vi "DELETE REASON.vi"(8 "error in (no error)":errorcluster, 11 "connection reference":T1) -> (0 "error out":errorcluster, 3 "connection reference out":T1)   [LabVIEW 2017]
uses:
  <vilib>/addons/database/Connection.llb/Conn ObjectReference.ctl
  <vilib>/addons/database/NI_Database_API.lvlib
panel:
  in  "CANCEL":bool
  in  "Select Serial Number":string(combo)
  in  "DELETE":bool
  # "Delete Reason"
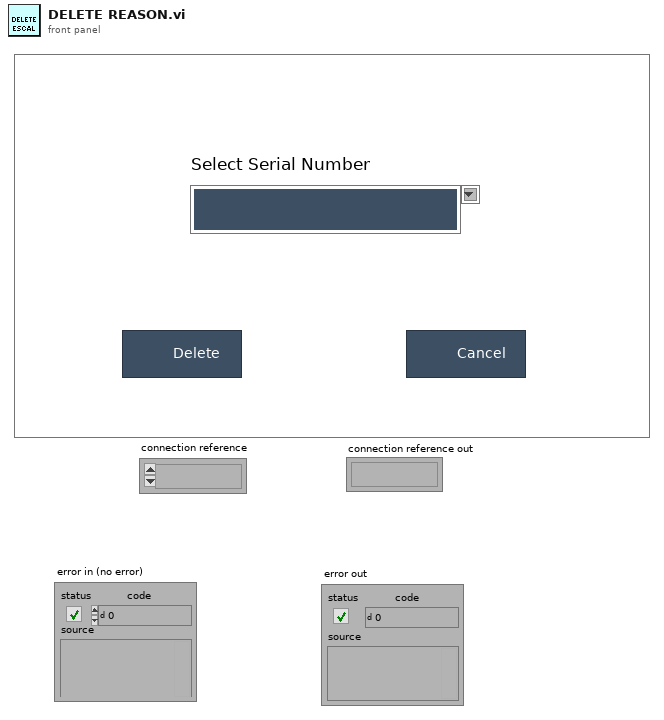
[diagram p1: front panel]
types:
  T1 = typedef "NI_Database_API.lvlib/Conn ObjectReference.ctl" = refnum<k1>
  T2 = enum32{"invalid app kind", "Development System", "Run Time System", "Student Edition", "Embedded LabVIEW", "Evaluation", "Custom"}
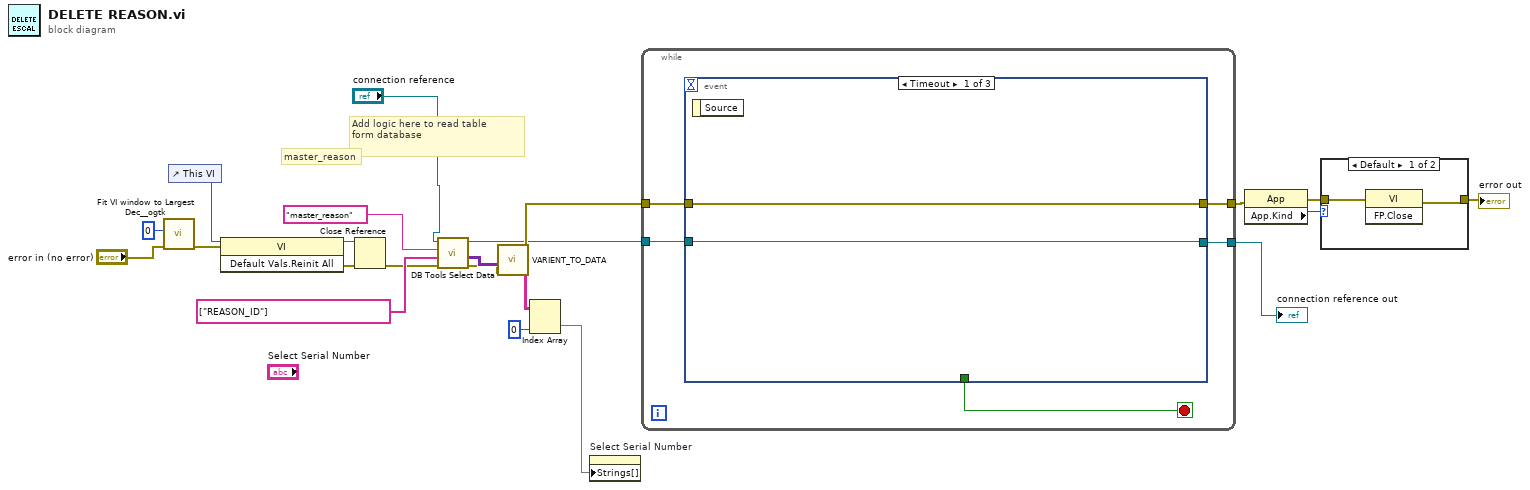
[diagram p0: block diagram]
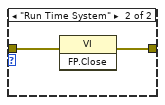
[diagram p2: hidden frame]
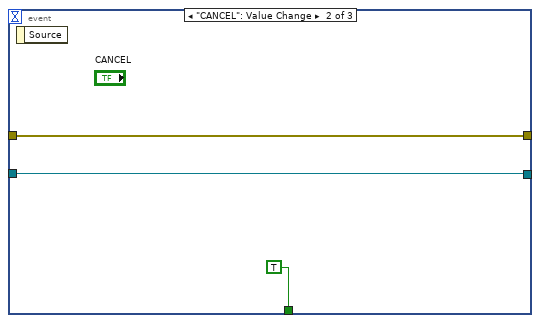
[diagram p3: hidden frame]
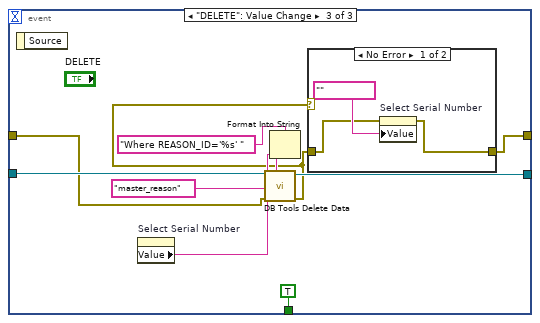
[diagram p4: hidden frame]
diagram:
  # "master_reason"
  # "Add logic here to read table\nform database"
  n1 = call <userlib>:"Fit VI window to Largest Dec__ogtk.vi"("error in (no error)"="error in (no error)", "border spacing (2 px)"=0) -> ("error out"=w2:errorcluster)  [unwired: 4 in, 1 out]
  n2 = control-ref of="This VI"() -> (w22:refnum<vi>)
  n3 = invoke class="VI" method="Default Vals.Reinit All"(reference=w22, error in=w2) -> (reference out=w20:refnum<vi>, error out=w21:errorcluster)  [unwired: 1 in, 1 out]
  n4 = Close Reference(reference=w20, error in (no error)=w21) -> (error out=w4:errorcluster)
  n5 = call <vilib>:"DB Tools Select Data.vi"("error in (no error)"=w4, "columns"=string[] ["REASON_ID"], "table"="master_reason", "connection reference"="connection reference") -> ("error out"=w14:errorcluster, "data"=w15:variant[][], "connection reference out"=w7:T1)  [unwired: 2 in]
  n6 = call "VARIENT_TO_DATA.vi"("data"=w15, "error in (no error)"=w14) -> ("Table"=w10:string[][], "error out"=w11:errorcluster)  [unwired: 7 in]
  n7 = Index Array(array=w10, index (col)=0 ("disabled index (col)")) -> (element=w8:string[])  [unwired: 1 in]
  n8 = property on="Select Serial Number" class="CmbBox"("Strings[]"=w8) -> ()  [unwired: 2 in, 2 out]
  n9 = while {
    tunnel: w11 -> [w27]
    tunnel: [w26] -> w16
    tunnel: w7 -> [w25]
    tunnel: [w24] -> w6
    stop <- w23 stop-if-true
    n10 = event shown="[0] Timeout" {
      selector: _ -> [_ _ _]
      dyn-events: _ -> [_ _ _]
      timeout: _ -> [_ _ _]
      tunnel: w27 -> [w29 w30 w41]
      tunnel: [w29 w30 w35] -> w26
      tunnel: w25 -> [w28 w31 w42]
      tunnel: [w28 w31 w40] -> w24
      tunnel: [_ TRUE TRUE] -> w23
      event Timeout {
        n11 = event-data() -> ()  [unwired: 1 in, 1 out]
      }
      event "CANCEL": Value Change {
        n12 = event-data() -> ()  [unwired: 1 in, 1 out]
      }
      event "DELETE": Value Change {
        n13 = event-data() -> ()  [unwired: 1 in, 1 out]
        n14 = property on="Select Serial Number" class="CmbBox"() -> ("Value"=w38:string)  [unwired: 2 in, 2 out]
        n15 = Format Into String(format string="Where REASON_ID='%s' " ("condition"), w38) -> (resulting string=w37:string)  [unwired: 2 in, 1 out]
        n16 = call <vilib>:"DB Tools Delete Data.vi"("condition"=w37, "error in (no error)"=w41, "table"="master_reason", "connection reference"=w42) -> ("error out"=w34:errorcluster, "connection reference out"=w40:T1)  [unwired: 6 in]
        n17 = case shown="No Error" w34 {
          tunnel: w34 -> [w43 w46]
          tunnel: [w44 w46] -> w35
          frame No Error {
            n18 = property on="Select Serial Number" class="CmbBox"(error in=w43, "Value"="") -> (error out=w44:errorcluster)  [unwired: 1 in, 1 out]
          }
          frame Error {
          }
        }
      }
    }
  }
  "connection reference out" <- w6
  n19 = property class="App"(error in=w16) -> (error out=w18:errorcluster, "App.Kind"=w19:T2)  [unwired: 1 in, 1 out]
  n20 = case shown="Default" w19 {
    tunnel: w18 -> [w48 w50]
    tunnel: [w47 w49] -> w17
    frame Default {
      n21 = invoke class="VI" method="FP.Close"(error in=w48) -> (error out=w47:errorcluster)  [unwired: 2 in, 2 out]
    }
    frame "Run Time System" {
      n22 = invoke class="VI" method="FP.Close"(error in=w50) -> (error out=w49:errorcluster)  [unwired: 2 in, 2 out]
    }
  }
  "error out" <- w17
